vi "GDSFile_CopyFolder.vi"(1 "source directory path":path, 2 "target directory path":path, 3 "Overwrite Existing Files? (FALSE)":bool, 5 "error in (no error)":errorcluster) -> (15 "dup target directory path":path, 19 "error out":errorcluster)   [LabVIEW 2020]
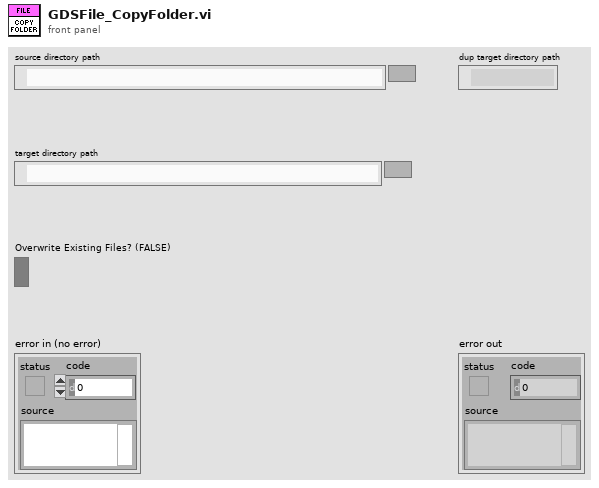
[diagram p1: front panel]
types:
  T1 = cluster{"Archive":bool, "Normal":bool, "Temporary":bool, "Compressed":bool, "Offline":bool, "Content Indexed":bool, "Encrypted (cannot set)":bool}
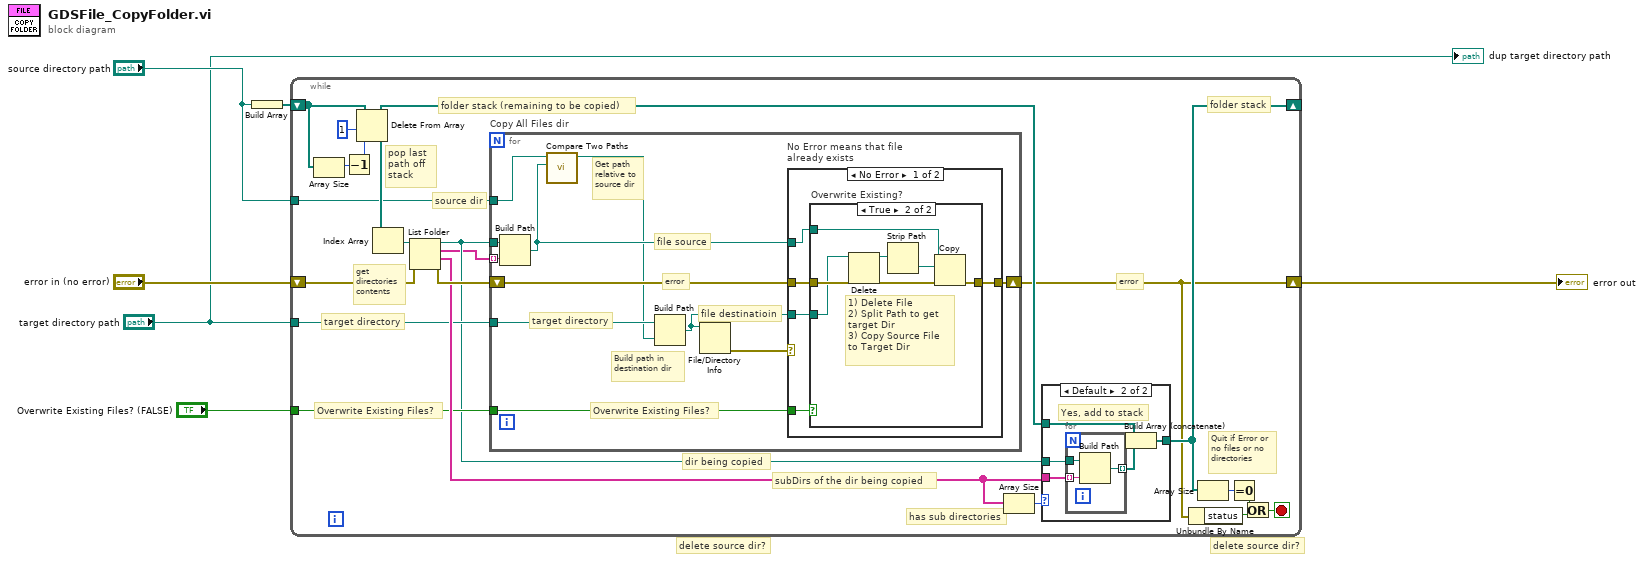
[diagram p0: block diagram]
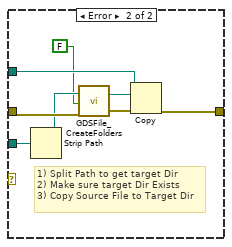
[diagram p4: hidden frame]
diagram:
  # "delete source dir?"
  # "delete source dir?"
  n1 = Build Array("source directory path") -> (w6:path[])
  n2 = while {
    shift-right: [w13] -> _
    shift-left: w6 -> [w16]
    shift-right: [w9] -> w1
    shift-left: "error in (no error)" -> [w17]
    tunnel: "source directory path" -> [w12]
    tunnel: "target directory path" -> [w11]
    tunnel: "Overwrite Existing Files? (FALSE)" -> [w10]
    stop <- w18 stop-if-true
    (unwired) T1 {"Archive"=FALSE, "Normal"=FALSE, "Temporary"=FALSE, "Compressed"=FALSE, "Offline"=FALSE, "Content Indexed"=FALSE, "Encrypted (cannot set)"=FALSE} ("FileAttribute")
    # "folder stack"
    # "error"
    # "Overwrite Existing Files?"
    # "target directory"
    # "subDirs of the dir being copied"
    # "dir being copied"
    # "folder stack (remaining to be copied)"
    # "source dir"
    # "get directories contents"
    # "pop last path off stack"
    # "Quit if Error or no files or no directories"
    # "has sub directories"
    n3 = Array Size(array=w16) -> (size(s)=w14:i32)
    n4 = Decrement(x=w14) -> (x-1=w15:i32)
    n5 = Delete From Array(array=w16, length=1 ("Length"), index=w15) -> (deleted portion=w27:path[], array with subset deleted=w22:path[])
    n6 = Index Array(array=w27) -> (element=w26:path)  [unwired: 1 in]
    n7 = List Folder(path=w26, error in=w17) -> (path out=w8:path, filenames=w7:string[], folder names=w23:string[], error out=w25:errorcluster)  [unwired: 2 in]
    n8 = for "Copy All Files dir" {
      shift-right: [w46] -> w9
      shift-left: w25 -> [w47]
      tunnel: w12 -> [w42]
      tunnel: w11 -> [w40]
      tunnel: w10 -> [w45]
      tunnel: w8 -> [w44]
      tunnel: w7 -> [w43] mode=indexing
      # "Overwrite Existing Files?"
      # "file destinatioin"
      # "file source"
      # "target directory"
      # "error"
      # "Build path in destination dir"
      # "Get path relative to source dir"
      n9 = Build Path(base path=w44, name or relative path=w43) -> (appended path=w41:path)
      n10 = call <vilib>:"Compare Two Paths.vi"("Path 2"=w41, "Path 1"=w42) -> ("Relative Path from 1 to 2"=w39:path)  [unwired: 6 in, 3 out]
      n11 = Build Path(base path=w40, name or relative path=w39) -> (appended path=w38:path)
      n12 = File/Directory Info(path=w38) -> (error out=w48:errorcluster)  [unwired: 1 in, 6 out]
      n13 = case "No Error means that file\nalready exists" shown="No Error" w48 {
        tunnel: w38 -> [w50 w67]
        tunnel: w41 -> [w49 w69]
        tunnel: w47 -> [w52 w64]
        tunnel: [w51 w68] -> w46
        tunnel: w45 -> [w53 _]
        frame No Error {
          n14 = case "Overwrite Existing?" shown="True" w53 {
            tunnel: w52 -> [w54 w59]
            tunnel: [w54 w61] -> w51
            tunnel: w50 -> [_ w57]
            tunnel: w49 -> [_ w60]
            frame False {
            }
            frame True {
              # "1) Delete File\n2) Split Path to get target Dir\n3) Copy Source File to Target Dir"
              n15 = Delete(path (use dialog)=w57, error in=w59) -> (deleted path=w56:path, error out=w58:errorcluster)  [unwired: 3 in, 1 out]
              n16 = Strip Path(path=w56) -> (stripped path=w55:path)  [unwired: 1 out]
              n17 = Copy(8:w58, 10:w55, 11:w60) -> (0:w61:errorcluster)  [unwired: 2 in, 2 out]
            }
          }
        }
        frame Error {
          # "1) Split Path to get target Dir\n2) Make sure target Dir Exists\n3) Copy Source File to Target Dir"
          n18 = Strip Path(path=w67) -> (stripped path=w63:path)  [unwired: 1 out]
          n19 = call "GDSFile_CreateFolders.vi"("Path"=w63, "Promt if folder\ndoes not exists?"=FALSE ("Promt if folder\ndoes not exists?"), "error in (no error)"=w64) -> ("PathOut"=w66:path, "error out"=w65:errorcluster)  [unwired: 12 in, 3 out]
          n20 = Copy(8:w65, 10:w66, 11:w69) -> (0:w68:errorcluster)  [unwired: 2 in, 2 out]
        }
      }
    }
    n21 = Array Size(array=w23) -> (size(s)=w24:i32)
    n22 = case shown="Default" w24 {
      tunnel: w8 -> [_ w31]
      tunnel: w23 -> [_ w32]
      tunnel: w22 -> [w29 w34]
      tunnel: [w29 w33] -> w13
      frame 0 {
      }
      frame Default {
        # "Yes, add to stack"
        n23 = for {
          tunnel: w31 -> [w37]
          tunnel: w32 -> [w36] mode=indexing
          tunnel: [w35] -> w30 mode=indexing
          n24 = Build Path(base path=w37, name or relative path=w36) -> (appended path=w35:path)
        }
        n25 = Build Array (concatenate)(w34, w30) -> (w33:path[])
      }
    }
    n26 = Unbundle By Name(w9) -> ("status"=w20:bool)
    n27 = Array Size(array=w13) -> (size(s)=w21:i32)
    n28 = Equal To 0?(x=w21) -> (x = 0?=w19:bool)
    n29 = Or(x=w19, y=w20) -> (x .or. y?=w18:bool)
  }
  "error out" <- w1
  "dup target directory path" <- "target directory path"
